vi "Set Device Properties.vi"(7 "CPU Assignment (-2)":i32=-2, 8 "error in (no error)":errorcluster, 9 "Decimation (1)":i32=1, 10 "VISA Name":string, 11 "Custom Device":refnum<k24>) -> (0 "error out":errorcluster, 3 "Custom Device Duplicate":refnum<k24>)   [LabVIEW 2010, in "RefMem PtByPt System Definition API.lvlib"]
doc: "Set the VISA name and Decimation of the custom device."
uses:
  RefMem PtByPt System Definition API.lvlib
  NationalInstruments.VeriStand.SystemDefinitionAPI
  <vilib>/NI Veristand/Custom Device API/Custom Device Path Data.ctl
  <vilib>/NI Veristand/Custom Device API/Custom Device Supported Target.ctl
  <vilib>/NI Veristand/Custom Device API/Path Specification.ctl
  <vilib>/NI Veristand/Custom Device API/Path Type.ctl
  <vilib>/NI Veristand/Custom Device API/Custom Device Execution Mode.ctl
  Custom Device/Controls/Global.vi
  Custom Device/RefMem PtByPt Custom Device.lvlib
  <vilib>/NI Veristand/Custom Device Offline API/Custom Device Offline API.lvlib
  <vilib>/NI Veristand/Custom Device API/Custom Device API.lvlib
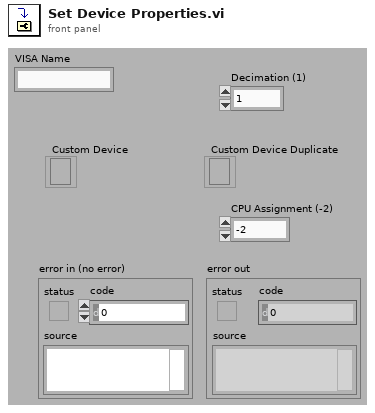
[diagram p1: front panel]
types:
  T1 = typedef "Custom Device API.lvlib/Custom Device Path Data.ctl" = cluster{"SupportedTarget":T2, "Source":T3, "RT Destination":path}
  T2 = typedef "Custom Device API.lvlib/Custom Device Supported Target.ctl" = enum16{"All", "PharLap", "VxWorks", "Windows", "PharLap & Windows", "PharLap & VxWorks", "VxWorks & Windows"}
  T3 = typedef "Custom Device API.lvlib/Path Specification.ctl" = cluster{"Path":path, "Type":T4}
  T4 = typedef "Custom Device API.lvlib/Path Type.ctl" = enum16{"Absolute", "To Base", "To Common Data Dir", "To Application Data Dir"}
  T5 = typedef "Custom Device API.lvlib/Custom Device Execution Mode.ctl" = enum16{"Asynchronous", "Inline HW Interface", "Inline Model Interface", "Inline Timing and Sync", "Asynchronous Timing and Sync"}
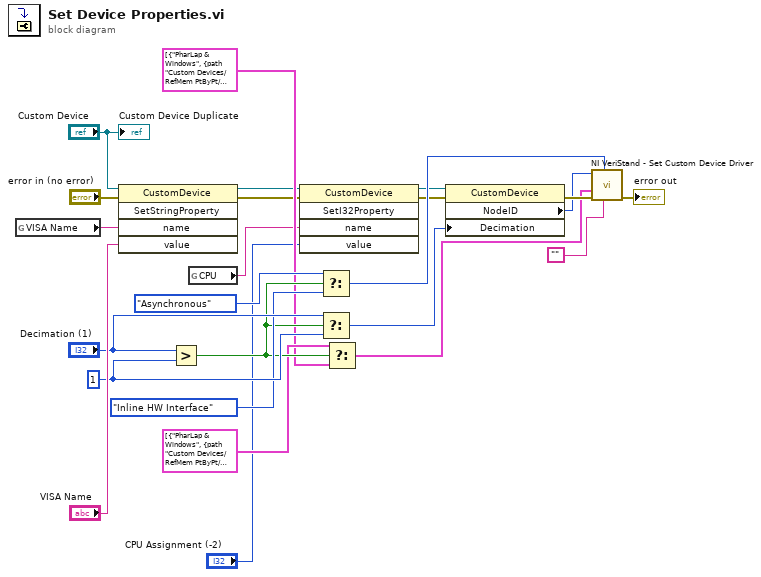
[diagram p0: block diagram]
diagram:
  w15 = u32 1 ("y")
  n1 = global read "Global.vi" "VISA Name"() -> (w22:string)
  n2 = invoke class="CustomDevice" method="SetStringProperty"(reference="Custom Device", error in="error in (no error)", "name"=w22, "value"="VISA Name") -> (reference out=w4:refnum<k24>, error out=w3:errorcluster)  [unwired: 1 in, 3 out]
  n3 = Greater?(x="Decimation (1)", y=w15) -> (0:w11:bool)
  n4 = global read "Global.vi" "CPU"() -> (w2:string)
  n5 = invoke class="CustomDevice" method="SetI32Property"(reference=w4, error in=w3, "name"=w2, "value"="CPU Assignment (-2)") -> (reference out=w6:refnum<k24>, error out=w5:errorcluster)  [unwired: 1 in, 3 out]
  n6 = Select(t=Custom_Device_Execution_Mode."Asynchronous" ("Execution mode"), s=w11, f=Custom_Device_Execution_Mode."Inline HW Interface" ("Execution mode")) -> (s? t:f=w8:T5)
  n7 = Select(t="Decimation (1)", s=w11, f=w15) -> (s? t:f=w16:u32)
  n8 = Select(t=T1[] [{"SupportedTarget"=enum."PharLap & Windows", "Source"={"Path"=path "Custom Devices/RefMem PtByPt/RefMem PtByPt Engine.llb/RefMem PtByPt RT Driver VI (Async).vi", "Type"=enum."To Common Data Dir"}, "RT Destination"=path "c:/ni-rt/VeriStand/Custom Devices/RefMem PtByPt/RefMem PtByPt Engine.llb/RefMem PtByPt RT Driver VI (Async).vi"}] ("Driver VI"), s=w11, f=T1[] [{"SupportedTarget"=enum."PharLap & Windows", "Source"={"Path"=path "Custom Devices/RefMem PtByPt/RefMem PtByPt Engine.llb/RefMem PtByPt RT Driver VI (Inline).vi", "Type"=enum."To Common Data Dir"}, "RT Destination"=path "c:/ni-rt/VeriStand/Custom Devices/RefMem PtByPt/RefMem PtByPt Engine.llb/RefMem PtByPt RT Driver VI (Inline).vi"}] ("Driver VI")) -> (s? t:f=w9:T1[])
  n9 = property class="CustomDevice"(reference=w6, error in=w5, "Decimation"=w16) -> (error out=w20:errorcluster, "NodeID"=w19:u64)  [unwired: 1 out]
  n10 = call <vilib>:"NI VeriStand - Set Custom Device Driver.vi"("Version"="", "Execution mode"=w8, "error in (no error)"=w20, "Driver VI"=w9, "Device Ref in"=w19) -> ("error out"=→"error out":errorcluster)  [unwired: 5 in, 1 out]
  "Custom Device Duplicate" <- "Custom Device"
